vi "QR_code_Check_St3.vi"(5 "Columns":string[](array[string]), 6 "Station 1 Bypass":bool, 7 "error in (no error)":errorcluster, 8 "replace %s":string, 9 "table":string, 10 "Refnum in":T1) -> (0 "error out":errorcluster, 1 "data":string[][](array[string]), 2 "FALSE healty":bool, 3 "Refnum out":T1, 4 "TRUE Duplication on Station 2":bool)   [LabVIEW 2017]
uses:
  <vilib>/addons/database/Connection.llb/Conn ObjectReference.ctl
  <vilib>/addons/database/NI_Database_API.lvlib
panel:
  out "resulting string":string
  out "TRUE no barcode Done on station 1":bool
  # "QR Code check St 3"
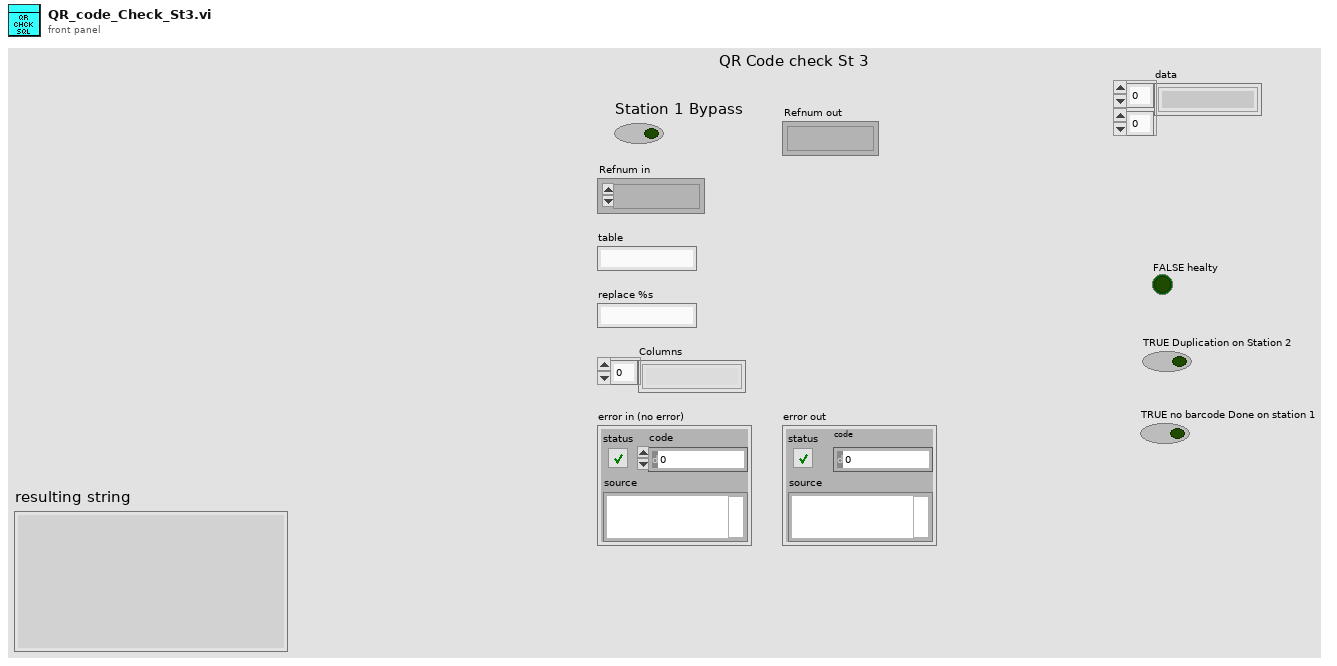
[diagram p1: front panel]
types:
  T1 = typedef "NI_Database_API.lvlib/Conn ObjectReference.ctl" = refnum<k1>
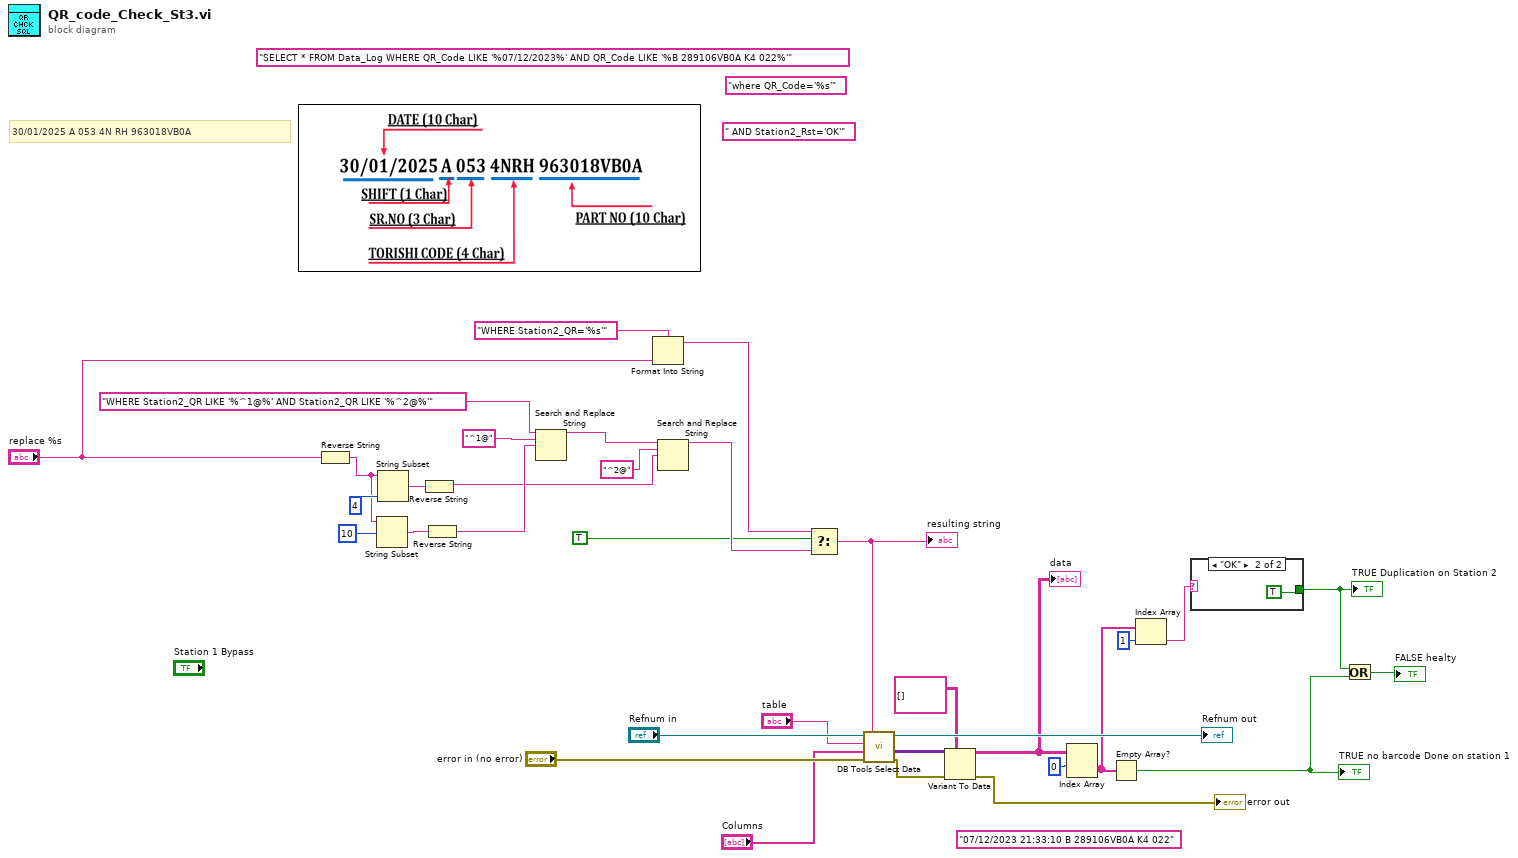
[diagram p0: block diagram]
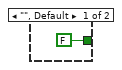
[diagram p2: hidden frame]
diagram:
  (unwired) "07/12/2023 21:33:10 B 289106VB0A K4 022" ("format string")
  (unwired) "SELECT * FROM Data_Log WHERE QR_Code LIKE '%07/12/2023%' AND QR_Code LIKE '%B 289106VB0A K4 022%'" ("format string")
  (unwired) "where QR_Code='%s'" ("format string")
  (unwired) " AND Station2_Rst='OK'" ("replace %s")
  # "30/01/2025 A 053 4N RH 963018VB0A"
  n1 = Reverse String(1:"replace %s") -> (0:w13:string)
  n2 = String Subset(string=w13, offset (0)=10) -> (substring=w12:string)  [unwired: 1 in]
  n3 = String Subset(string=w13, length (rest)=4 ("offset (0)")) -> (substring=w14:string)  [unwired: 1 in]
  n4 = Reverse String(1:w14) -> (0:w6:string)
  n5 = Reverse String(1:w12) -> (0:w7:string)
  n6 = Search and Replace String(input string="WHERE Station2_QR LIKE '%^1@%' AND Station2_QR LIKE '%^2@%'" ("format string"), search string="^1@", replace string=w7) -> (result string=w10:string)  [unwired: 5 in, 3 out]
  n7 = Format Into String(format string="WHERE Station2_QR='%s'", "replace %s") -> (resulting string=w3:string)  [unwired: 2 in, 1 out]
  n8 = Search and Replace String(input string=w10, search string="^2@", replace string=w6) -> (result string=w4:string)  [unwired: 5 in, 3 out]
  n9 = Select(t=w3, s=TRUE, f=w4) -> (s? t:f=w2:string)
  "resulting string" <- w2
  n10 = call <vilib>:"DB Tools Select Data.vi"("condition"=w2, "error in (no error)"="error in (no error)", "columns"="Columns", "table"="table", "connection reference"="Refnum in") -> ("error out"=w24:errorcluster, "data"=w26:variant[][], "connection reference out"=→"Refnum out":T1)  [unwired: 1 in]
  n11 = Variant To Data(error in=w24, type=string[][] [], Variant=w26) -> (data=w25:string[][], error out=→"error out":errorcluster)
  "data" <- w25
  n12 = Index Array(array=w25, index (row)=0) -> (element=w22:string[])  [unwired: 1 in]
  n13 = Empty Array?(array=w22) -> (empty?=w19:bool)
  "TRUE no barcode Done on station 1" <- w19
  n14 = Index Array(array=w22, index=1 ("index (row)")) -> (element=w21:string)
  n15 = case shown="\"OK\"" w21 {
    tunnel: [FALSE TRUE] -> w18
    frame "", Default {
    }
    frame "OK" {
    }
  }
  "TRUE Duplication on Station 2" <- w18
  n16 = Or(x=w18, y=w19) -> (x .or. y?=→"FALSE healty":bool)
